vi "16bit-signed-to-16bit-unsigned.vi"(11 "Image Array":i32[][](array[numeric])) -> (3 "Image Array out":i32[][](array[numeric]))   [LabVIEW 2014]
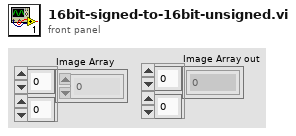
[diagram p1: front panel]
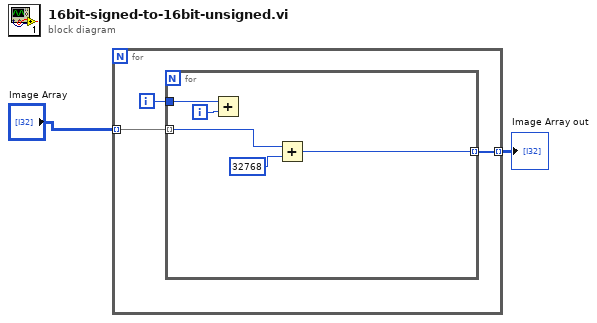
[diagram p0: block diagram]
diagram:
  n1 = for {
    tunnel: "Image Array" -> [w5] mode=indexing
    tunnel: [w3] -> w1 mode=indexing
    i -> [w4]
    n2 = for {
      tunnel: w5 -> [w8] mode=indexing
      tunnel: w4 -> [w10]
      tunnel: [w6] -> w3 mode=indexing
      i -> [w9]
      n3 = Add(x=w10, y=w9) -> ()  [unwired: 1 out]
      n4 = Add(x=w8, y=32768) -> (x+y=w6:i32)
    }
  }
  "Image Array out" <- w1
